vi "Send stop routine.vi"(8 "error in (no error)":errorcluster, 11 "Queue in":refnum<queue>) -> (0 "error out":errorcluster)   [LabVIEW 2020]
uses:
  Message Queue/Message Cluster.ctl
  Message Queue/Enqueue Message (Single).vi
  Message Queue/Message Queue.lvlib
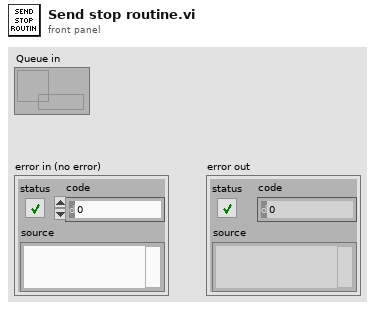
[diagram p1: front panel]
types:
  T1 = enum8{"Enabled", "Disabled", "Disabled and Grayed Out"}[]
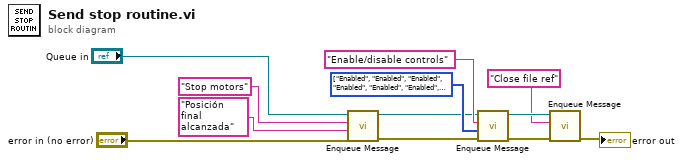
[diagram p0: block diagram]
diagram:
  w8 = T1 [enum."Enabled", enum."Enabled", enum."Enabled", enum."Enabled", enum."Enabled", enum."Enabled", enum."Enabled", enum."Enabled", enum."Disabled and Grayed Out", enum."Enabled", enum."Enabled"] items=["Enabled", "Disabled", "Disabled and Grayed Out"] ("Disabled")
  n1 = call-poly "Enqueue Message.vi"("error in (no error)"="error in (no error)", "Message Data"="Posición final alcanzada", "Message"="Stop motors", "Message Queue"="Queue in") -> ("error out"=w5:errorcluster, "dup Message Queue"=w6:refnum<queue>)  [unwired: 6 in]
  n2 = call-poly "Enqueue Message.vi"("error in (no error)"=w5, "Message Data"=w8, "Message"="Enable/disable controls", "Message Queue"=w6) -> ("error out"=w9:errorcluster, "dup Message Queue"=w12:refnum<queue>)  [unwired: 6 in]
  n3 = call-poly "Enqueue Message.vi"("error in (no error)"=w9, "Message"="Close file ref", "Message Queue"=w12) -> ("error out"=→"error out":errorcluster)  [unwired: 7 in, 1 out]
